vi "Robot Global Data.vi"() -> ()   [LabVIEW 2015]
doc: "This global VI can contain as many global variables as you need. Place a control on the panel, give it a good name. To read or write to it from a VI, drag the icon to the diagram of that VI. You can also drag from the project. Click on the node to change which global you access. You shouldn't have multiple locations writing to a global or it will cause a race-condition."
uses:
  <vilib>/Rock Robotics/WPI/Camera/WPI_CameraImageSize.ctl
  <vilib>/Rock Robotics/WPI/DriverStation/WPI_DriverStationRobotMode2.ctl
  Common Code/Auton Command Cluster.ctl
  Common Code/Drivetrain Status Cluster.ctl
  Common Code/Drivetrain Modes.ctl
  Common Code/Dist Drive Status.ctl
  Common Code/Dashboard Communication/Dashboard Display Data.ctl
  Common Code/Auton File Lists.ctl
  Common Code/Encoder Values Super Cluster.ctl
  Common Code/Encoder Values.ctl
  Common Code/IMU Data.ctl
  navX.Library.v2/navX Library v2/TypeDefs/Flags/Z900_navX_Flags_CalibrationStatusTypeDef.ctl
  navX.Library.v2/navX Library v2/TypeDefs/Flags/Z900_navX_Flags_OpStatusTypeDef.ctl
  Common Code/Power and Diagnostic Data.ctl
  Common Code/Utilities/PDP Data.ctl
  Common Code/Utilities/PCM Data.ctl
  Common Code/Intake Status Cluster.ctl
  Common Code/Intake Mode.ctl
  Common Code/Intake Commands.ctl
  Common Code/Ultrasonic Data.ctl
  Common Code/Major Loop Times.ctl
  Common Code/Catapult/Catapult Status Cluster.ctl
  Common Code/Catapult/Catapult Modes.ctl
  Common Code/Catapult/Catapult Auto Commands.ctl
  Common Code/Catapult/Shoot Mode.ctl
  Common Code/Dashboard Communication/Dashboard Control Data.ctl
  Common Code/Encoder Control.ctl
  Common Code/Drivetrain Settings.ctl
  Common Code/Goal Vision Packet.ctl
  Common Code/Dashboard Drivetrain Command.ctl
  Common Code/Drivetrain Vision.ctl
  Common Code/Ball Tracking Command Cluster.ctl
  Common Code/Ball Vision Packet.ctl
  Common Code/Tracking Mode.ctl
  Common Code/Intake Presets.ctl
  Common Code/Drivetrain Output Range.ctl
  Common Code/IntakeEcoderControl.ctl
  Common Code/Enabled Systems.ctl
  Common Code/Autonomous Presets.ctl
  Common Code/Auto Shift Cluster.ctl
  Common Code/Catapult/Catapult Presets.ctl
  Common Code/Climb Presets.ctl
  Common Code/Drivetrain Commands.ctl
  Common Code/Manual Shoot.ctl
  Common Code/Intake Commands Cluster.ctl
  Common Code/Manual Intake Commands.ctl
  Common Code/Keyboard Packet.ctl
  Common Code/Catapult/Catapult Command Cluster.ctl
  navX.Library.v2/navX Library v2/navX Library v2.lvlib
panel:
  in  "Catapult Status Cluster":T1={"Shoot? "=FALSE, "Mode"=enum."Auto", "States"=enum."Shoot", "Shoot Mode"=enum."Outer", "Override IR "=FALSE, "Ball Loaded? "=FALSE, "High Pressure?"=FALSE, "Enough Pressure? "=enum."NO ", "high 1"=FALSE, "high 2 "=FALSE, "high 3"=FALSE, "high 4"=FALSE, "Jank Boi"=FALSE, "Ball Security"=FALSE, "Flashlight "=FALSE}
  in  "Catapult Command Cluster":T5={"States"=enum."Shoot", "Mode"=enum."Auto", "Override IR"=FALSE, "Shoot Mode"=enum."Outer", "Ball Loaded?"=FALSE, "High Pressure?"=FALSE, "Shoot?"=FALSE, "Flashlight "=FALSE}
  in  "Goal Vision Packet":T6
  in  "Auton Line Number":i32
  out "Current Position":dbl
  out "Backward Intake Tripped?":bool
  out "Forward Intake Tripped?":bool
  in  "Zero Intake?":bool
  out "Auton File Loop Timer":u32
  out "US Loop Timer":u32
  out "Intake Loop Timer":u32
  out "Shooter Loop Timer":u32
  out "DT Loop Timer":u32
  out "Ultrasonic Data":T7
  in  "Keyboard Cluster":T8
  in  "Intake Status Cluster":T9={"Roller Power"=0.0, "Angle Power"=0.0, "Intake Mode"=enum."Auto", "Rollers Active?"=FALSE, "Current Height"=0.0, "Target Height"=0.0, "Encoder Raw Position"=0.0, "Forward Tripped?"=FALSE, "Backward Tripped?"=FALSE, "Override IR?"=FALSE, "Intake State"=enum."Zero"}
  out "Is IMU Reset?":bool
  in  "Reset IMU":bool
  in  "Boolean":bool
  in  "Intake Commands Cluster":T12={"Intake Commands"=enum."Load", "Intake Mode"=enum."Auto", "Override IR"=FALSE}
  in  "Manual Intake Commands":T13
  in  "Queue File Names":string[](array[string])
  in  "NavX Opened":bool
  in  "IMU Yaw Zero":dbl
  in  "IMU Roll Zero":dbl
  in  "IMU Pitch Zero":dbl
  in  "Manual Shoot":T14
  out "IMU Data":T15 {"OP Status" items=["INITIALIZING", "SELFTEST_IN_PROGRESS", "ERROR", "IMU_AUTOCAL_IN_PROGRESS", "NORMAL"]; "Calibration Status" items=["IMU_CAL_STATE_MASK"=3, "IMU_CAL_STATE_INPROGRESS"=0, "IMU_CAL_STATE_ACCUMULATE"=1, "IMU_CAL_STATE_COMPLETE"=2]}
  in  "Right Pot 0":dbl
  in  "Left Pot 0":dbl
  out "Encoder Values":T18
  in  "Dashboard Drivetrain Command":T20
  out "General Scripts":string
  in  "Auton File Lists":T22
  in  "Current Auton Command Data":T23
  in  "Dashboard Packet":T24={"Encoder Control"={"Right Tick Constant"=0.0, "Left Tick Constant"=0.0, "Reset?"=FALSE, "Y Dist"={"PID gains"={"proportional gain (Kc)"=0.0, "integral time (Ti, min)"=0.0, "derivative time (Td, min)"=0.0}}, "Y Stop Thresh"=0.0, "Y Stop Speed"=0.0}, "Steer PID output"={"output high"=0.0, "output low"=0.0}, " Steer PID gains"={"proportional gain (Kc)"=0.0, "integral time (Ti, min)"=0.0, "derivative time (Td, min)"=0.0}, "Drivetrain Settings"={"Gyro Tolerance"=0.0, "Throttle Ramp (ms)"=0.0, "Kv"=0.0, "Ka"=0.0, "Feed Forward P"=0.0, "Feed Forward D"=0.0, "Goal Vision PID gains"={"proportional gain (Kc)"=1.0, "integral time (Ti, min)"=0.01, "derivative time (Td, min)"=0.0}, "Goal Detection Window"=0.0, "Creep Rate"=0.0, "Vision Throttle Threshold"=0.0, "Min Turn Output"=0.0, "Left Batter Angle"=0.0, "Right Batter Angle"=0.0}, "Vision Packet"={"Distance"=0.0, "Center X"=0.0, "Center Y"=0.0, "Found Target?"=FALSE, "Robot Center"=0.0, "Angle"=0.0}, "Dashboard Drivetrain Command"={"Drivetrain Vision"={"Goal Window"=0.0, "Ball Window"=0.0}}, "Info/Command Cluster"={"Distance to Ball"=0.0, "Desired Angle"=0.0, "Command"=enum."Turn to Ball", "Pixels from Center"=0.0}, "Ball Vision Packet"={"Ball Detected?"=FALSE, "Distance to Ball"=0.0, "Desired Angle"=0.0, "Pixels from Center"=0.0, "Tracking mode"=enum."Turn to Ball"}, "Intake Presets"={"Intake Speed"=0.0, "Outake Speed"=0.0, "Angle Speed"=0.0, "Angle Tolerance"=0.0, "Encoder Scale"=0.0, "Load Height"=0.0, "Output Range"={"output high"=0.0, "output low"=0.0}, "MaxCurrent"=0.0, "Idle Height"=0.0, "Max Height"=0.0, "Reset Encoders?"=FALSE, "PID gains"={"proportional gain (Kc)"=0.0, "integral time (Ti, min)"=0.0, "derivative time (Td, min)"=0.0}, "Drop Low Height "=0.0, "Rotation Power Max/Min"=0.0, "Reset Delay"=0.0}, "Intake Encoder Control"={"Arm Tick Constant"=0.0, "Reset?"=FALSE, "Y Dist"={"PID gains"={"proportional gain (Kc)"=0.0, "integral time (Ti, min)"=0.0, "derivative time (Td, min)"=0.0}}, "Y Stop Thresh"=0.0, "Y Stop Speed"=0.0}, "Goal Output Range"={"output high"=0.0, "output low"=0.0}, "Enabled Systems"={"Shoot"=TRUE, "Intake"=TRUE, "DT"=TRUE, "Gyro"=TRUE, "100ms"=TRUE, "US"=TRUE}, "Auton Presets"={"Pitch Limit"=0.0, "Roll Limit"=0.0, "Start Position"=0.0, "Cross Position"=0.0}, "Pressure M"=0.0, "Pressure B"=0.0, "Vision Timeout"=0.0, "Auto-Shift"={"Delay"=0.0, "Speed Thresh"=0.0, "Upshift Accel"=0.0, "Upshift Throttle"=0.0, "Upshift Throttle Accel"=0.0, "Downshift Throttle"=0.0, "Downshift Throttle Accel"=0.0, "Pressure Threshold"=0.0}, "Catapult Setpoints"={"Intake Danger Height"=0.0, "Ball Security Delay "=0.0, "High PSI Minimum"=0.0, "Shot Finish Delay"=0.0, "Low PSI Minimum"=0.0, "Idle Ball Security Wait "=0.0}, "Climb Presets"={"Winch Speed"=0.0}} {"Intake Presets"."Reset Delay" format="%#_7g"; "Intake Presets"."Rotation Power Max/Min" format="%#_7g"; "Intake Presets"."Drop Low Height" format="%#_7g"; "Intake Presets"."Max Height" format="%#_7g"; "Drivetrain Settings"."Goal Vision PID gains"."derivative time (Td, min)" format="%.3f"; "Drivetrain Settings"."Goal Vision PID gains"."integral time (Ti, min)" format="%.3f"; "Drivetrain Settings"."Goal Vision PID gains"."proportional gain (Kc)" format="%.3f"}
  out "Driver Station IP":u32
  in  "Auton File Index":i32
  in  "Auton Field Index":i32
  out "Dashboard Status Data":T38={"Auton Command Cluster"={"Command ID"=0, "maxTime"=0.0, "Y Distance"=0.0, "Heading"=0.0, "Throttle"=0.0, "Async"=0.0, "Velocity"=0.0, "Acceleration"=0.0, "To"=0.0, "Condition"=0.0, "Shot Type"=0.0, "Left RPM"=0.0, "Override RPM"=0, "Override Angle"=0, "Right RPM"=0.0, "Angle"=0.0, "Intake Mode"=0, "Intake Cmd"=0, "Intake O"=0, "Eject O"=0, "Angle O"=0, "Arm O"=0, "Intake Speed"=0.0, "Eject Speed"=0.0, "Arm Angle"=0.0, "Arm Speed"=0.0, "Intake?"=0, "Eject?"=0, "Left"=0.0, "Right"=0.0, "Pivot Speed"=0.0, "Y Dist"=0.0, "Position"=0.0, "Desired Position"=0, "Shooter Mode"=0.0, "Shooter Command"=0.0, "Shoot?"=0.0, "Shoot mode"=0.0}, "Auton File Lists"={"Current Queue"="", "General Scripts"="", "Defense Scripts"="", "Movement Scripts"=""}, "Drivetrain Status Cluster"={"Modes"=enum."Manual", "Y (Throttle)"=0.0, "X (Steer)"=0.0, "Gyro In Range?"=FALSE, "Distance Drive Finished?"=FALSE, "Stop Eject Lockout"=FALSE, "Dist Drive Status"={"Y In Range"=FALSE, "X In Range"=FALSE, "Gyro In Range"=FALSE, "Y Dist"=0.0, "X Dist"=0.0, "Gyro"=0.0}, "Y Target"=0.0, "Heading Target"=0.0, "Vision Target Aligned?"=FALSE}, "Encoder Values"={"Left Encoder"={"Distance"=0.0, "Speed"=0.0, "Ticks"=0.0}, "Right Encoder"={"Distance"=0.0, "Speed"=0.0, "Ticks"=0.0}}, "IMU Data"={"Pitch"=0.0, "Roll"=0.0, "Yaw"=0.0, "Data Valid?"=FALSE, "Temp"=0.0, "MOVING"=FALSE, "YAW_STABLE"=FALSE, "Accel X"=0.0, "Accel Y"=0.0, "Accel Z"=0.0, "Accel Magnitude"=0.0, "Pitch Rate"=0.0, "Roll Rate"=0.0, "Yaw Rate"=0.0, "NavX Opened?"=FALSE, "Calibration Status"=0, "OP Status"=0}, "Power and Diagnostic Data"={"PDP Data"={"Battery Voltage"=0.0, "Temperature (degrees C)"=0.0, "Internal Battery R (Ohms)"=0.0, "Energy (J)"=0.0, "Power (W)"=0.0, "Total Current (A)"=0.0, "Battery Voltage Fault"=FALSE, "Temperature Fault"=FALSE, "Hardware Fault"=FALSE, "Currents"={"[0]"=0.0, "[1]"=0.0, "[2]"=0.0, "[3]"=0.0, "[4]"=0.0, "[5]"=0.0, "[6]"=0.0, "[7]"=0.0, "[8]"=0.0, "[9]"=0.0, "[10]"=0.0, "[11]"=0.0, "[12]"=0.0, "[13]"=0.0, "[14]"=0.0, "[15]"=0.0}, "Current Faults"={"[0]"=FALSE, "[1]"=FALSE, "[2]"=FALSE, "[3]"=FALSE, "[4]"=FALSE, "[5]"=FALSE, "[6]"=FALSE, "[7]"=FALSE, "[8]"=FALSE, "[9]"=FALSE, "[10]"=FALSE, "[11]"=FALSE, "[12]"=FALSE, "[13]"=FALSE, "[14]"=FALSE, "[15]"=FALSE}}, "PCM Data"={"Compressor Fault"=FALSE, "Solenoid Fault"=FALSE, "Compressor Enabled"=FALSE, "Hardware Fault"=FALSE, "Compressor Current"=0.0}, "roboRIO input voltage (V)"=0.0, "roboRIO input current (A)"=0.0, "3.3V Rail Short"=FALSE, "5 V Rail Short"=FALSE, "6 V Rail Short"=FALSE, "roboRIO Brownout"=FALSE, "Outputs Enabled?"=FALSE}, "Gyro"=0.0, "Intake Status Cluster"={"Roller Power"=0.0, "Angle Power"=0.0, "Intake Mode"=enum."Auto", "Rollers Active?"=FALSE, "Current Height"=0.0, "Target Height"=0.0, "Encoder Raw Position"=0.0, "Forward Tripped?"=FALSE, "Backward Tripped?"=FALSE, "Override IR?"=FALSE, "Intake State"=enum."Zero"}, "Ultrasonic Data"={"Left Ultrasonic"=0.0, "Right Ultrasonic"=0.0}, "Loop Times"={"DT Loop Timer"=0, "Shooter Loop Timer"=0, "Intake Loop Timer"=0, "US Loop Timer"=0, "Auton File Loop Timer"=0}, "Pressure"=0.0, "Pressure Voltage"=0.0, "Auton Line Number"=0, "Catapult Status Cluster "={"Shoot? "=FALSE, "Mode"=enum."Auto", "States"=enum."Shoot", "Shoot Mode"=enum."Outer", "Override IR "=FALSE, "Ball Loaded? "=FALSE, "High Pressure?"=FALSE, "Enough Pressure? "=enum."NO ", "high 1"=FALSE, "high 2 "=FALSE, "high 3"=FALSE, "high 4"=FALSE, "Jank Boi"=FALSE, "Ball Security"=FALSE, "Flashlight "=FALSE}, "Forward Tripped?"=FALSE, "Backward Tripped?"=FALSE} {"IMU Data"."OP Status" items=["INITIALIZING", "SELFTEST_IN_PROGRESS", "ERROR", "IMU_AUTOCAL_IN_PROGRESS", "NORMAL"]; "IMU Data"."Calibration Status" items=["IMU_CAL_STATE_MASK"=3, "IMU_CAL_STATE_INPROGRESS"=0, "IMU_CAL_STATE_ACCUMULATE"=1, "IMU_CAL_STATE_COMPLETE"=2]}
  in  "Auton File Build Loops":i32
  in  "Auton File Queue":path[](array[path])
  in  "Auton Command Array":T23[](array[typedef])
  out "Drivetrain Status Cluster":T39={"Modes"=enum."Manual", "Y (Throttle)"=0.0, "X (Steer)"=0.0, "Gyro In Range?"=FALSE, "Distance Drive Finished?"=FALSE, "Stop Eject Lockout"=FALSE, "Dist Drive Status"={"Y In Range"=FALSE, "X In Range"=FALSE, "Gyro In Range"=FALSE, "Y Dist"=0.0, "X Dist"=0.0, "Gyro"=0.0}, "Y Target"=0.0, "Heading Target"=0.0, "Vision Target Aligned?"=FALSE}
  in  "Drivetrain Command Cluster":T46={"Y Power"=0.0, "Turn Power"=0.0, "Modes"=enum."Manual", "Heading Target"=0.0, "X Max Speed"=0.0, "Y Max Speed"=0.0, "X Min Speed"=0.0, "Y Min Speed"=0.0, "Y Target"=0.0, "Max Accel"=0.0, "Max Velocity"=0.0, "Pivot Speed"=0.0}
  in  "Robot Mode":T47
  in  "image size":T48=enum."320x240"
  in  "Enable Vision":bool
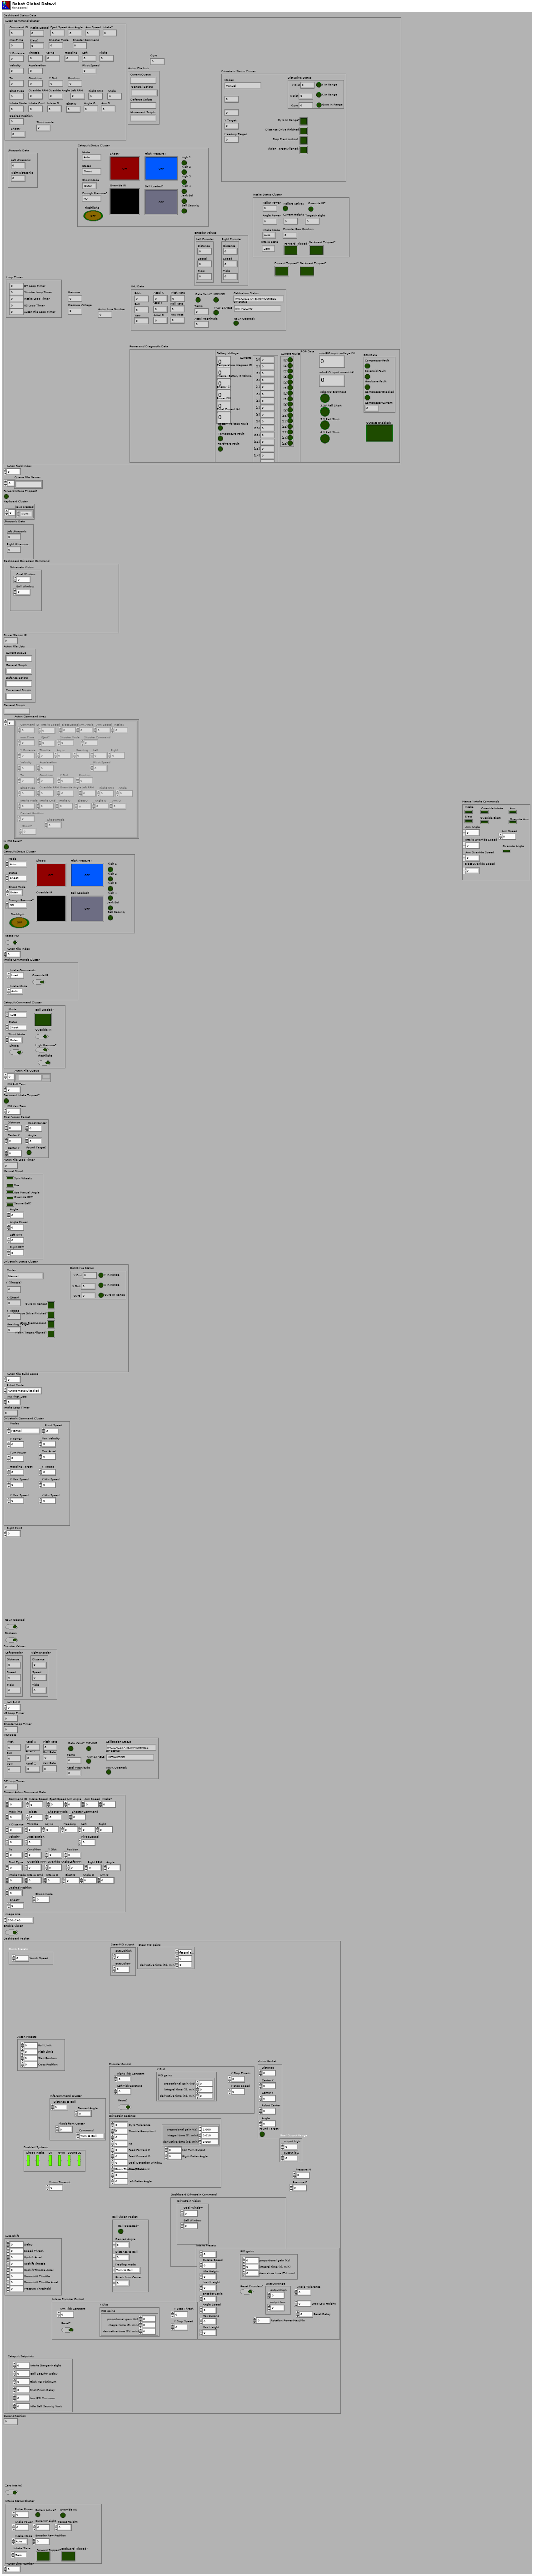
[diagram p1: front panel]
types:
  T1 = typedef "Catapult Status Cluster.ctl" = cluster{"Shoot? ":bool, "Mode":T2, "States":T3, "Shoot Mode":T4, "Override IR ":bool, "Ball Loaded? ":bool, "High Pressure?":bool, "Enough Pressure? ":enum16{"NO ", "Low Pressure", "High Pressure "}, "high 1":bool, "high 2 ":bool, "high 3":bool, "high 4":bool, "Jank Boi":bool, "Ball Security":bool, "Flashlight ":bool}
  T2 = typedef "Catapult Modes.ctl" = enum16{"Auto"}
  T3 = typedef "Catapult Auto Commands.ctl" = enum16{"Idle", "Warmup", "Shoot"}
  T4 = typedef "Shoot Mode.ctl" = enum16{"Outer", "Batter"}
  T5 = typedef "Catapult Command Cluster.ctl" = cluster{"States":T3, "Mode":T2, "Override IR":bool, "Shoot Mode":T4, "Ball Loaded?":bool, "High Pressure?":bool, "Shoot?":bool, "Flashlight ":bool}
  T6 = typedef "Goal Vision Packet.ctl" = cluster{"Distance":dbl, "Center X":dbl, "Center Y":dbl, "Found Target?":bool, "Robot Center":dbl, "Angle":dbl}
  T7 = typedef "Ultrasonic Data.ctl" = cluster{"Left Ultrasonic":dbl, "Right Ultrasonic":dbl}
  T8 = typedef "Keyboard Packet.ctl" = cluster{"keys pressed":enum16{"0", "1", "2", "3", "4", "5", "6", "7", "8", "9", "A", "B", "C", "D", "E", "F", "G", "H", "I", "J", "K", "L", "M", "N", "O", "P", "Q", "R", "S", "T", "U", "V", "W", "X", "Y", "Z", "F1", "F2", "F3", "F4", "F5", "F6", "F7", "F8", "F9", "F10", "F11", "F12", "F13", "F14", "F15", "ADD", "BACK", "BACKSLASH", "CAPITAL", "COMMA", "DECIMAL", "DELETE", "DIVIDE", "DOWN", "END", "EQUALS", "ESCAPE", "GRAVE (`)", "HOME", "INSERT", "LBRACKET", "LCONTROL", "LEFT", "L ALT", "LSHIFT", "LWIN", "MINUS", "MULTIPLY", "NEXT", "NUMLOCK", "NUMPAD_0", "NUMPAD_1", "NUMPAD_2", "NUMPAD_3", "NUMPAD_4", "NUMPAD_5", "NUMPAD_6", "NUMPAD_7", "NUMPAD_8", "NUMPAD_9", "PAUSE", "PERIOD", "PRIOR (PG UP)", "RBRACKET", "RCONTROL", "RETURN", "RIGHT", "R ALT", "RSHIFT", "RWIN", "SCROLL", "SEMICOLON", "SLASH", "SPACE", "SUBTRACT", "TAB", "UP", "ENTER (num pad)", "' (quote)"}[]}
  T9 = typedef "Intake Status Cluster.ctl" = cluster{"Roller Power":dbl, "Angle Power":dbl, "Intake Mode":T10, "Rollers Active?":bool, "Current Height":dbl, "Target Height":dbl, "Encoder Raw Position":dbl, "Forward Tripped?":bool, "Backward Tripped?":bool, "Override IR?":bool, "Intake State":T11}
  T10 = typedef "Intake Mode.ctl" = enum16{"Manual", "Safe", "Auto"}
  T11 = typedef "Intake Commands.ctl" = enum16{"Zero", "Unload", "Load", "Drop low", "Idle"}
  T12 = typedef "Intake Commands Cluster.ctl" = cluster{"Intake Commands":T11, "Intake Mode":T10, "Override IR":bool}
  T13 = typedef "Manual Intake Commands.ctl" = cluster{"Intake":bool, "Eject":bool, "Arm Angle":dbl, "Intake Override Speed":dbl, "Arm Override Speed":dbl, "Arm Speed":dbl, "Override Intake":bool, "Override Eject":bool, "Eject Override Speed":dbl, "Arm":bool, "Override Arm":bool, "Override Angle":bool}
  T14 = typedef "Manual Shoot.ctl" = cluster{"Spin Wheels":bool, "Fire":bool, "Angle":dbl, "Angle Power":dbl, "Use Manual Angle":bool, "Override RPM":bool, "Left RPM":dbl, "Right RPM":dbl, "Secure Ball?":bool}
  T15 = typedef "IMU Data.ctl" = cluster{"Pitch":sgl, "Roll":sgl, "Yaw":sgl, "Data Valid?":bool, "Temp":sgl, "MOVING":bool, "YAW_STABLE":bool, "Accel X":sgl, "Accel Y":sgl, "Accel Z":sgl, "Accel Magnitude":sgl, "Pitch Rate":sgl, "Roll Rate":sgl, "Yaw Rate":sgl, "NavX Opened?":bool, "Calibration Status":T16, "OP Status":T17}
  T16 = typedef "navX Library v2.lvlib/Z900_navX_Flags_CalibrationStatusTypeDef.ctl" = u8
  T17 = typedef "navX Library v2.lvlib/Z900_navX_Flags_OpStatusTypeDef.ctl" = u8
  T18 = typedef "Encoder Values Super Cluster.ctl" = cluster{"Left Encoder":T19, "Right Encoder":T19}
  T19 = typedef "Encoder Values.ctl" = cluster{"Distance":dbl, "Speed":dbl, "Ticks":dbl}
  T20 = typedef "Dashboard Drivetrain Command.ctl" = cluster{"Drivetrain Vision":T21}
  T21 = typedef "Drivetrain Vision.ctl" = cluster{"Goal Window":dbl, "Ball Window":dbl}
  T22 = typedef "Auton File Lists.ctl" = cluster{"Current Queue":string, "General Scripts":string, "Defense Scripts":string, "Movement Scripts":string}
  T23 = typedef "Auton Command Cluster.ctl" = cluster{"Command ID":i32, "maxTime":dbl, "Y Distance":dbl, "Heading":dbl, "Throttle":dbl, "Async":dbl, "Velocity":dbl, "Acceleration":dbl, "To":dbl, "Condition":dbl, "Shot Type":dbl, "Left RPM":dbl, "Override RPM":i32, "Override Angle":i32, "Right RPM":dbl, "Angle":dbl, "Intake Mode":i32, "Intake Cmd":i32, "Intake O":i32, "Eject O":i32, "Angle O":i32, "Arm O":i32, "Intake Speed":dbl, "Eject Speed":dbl, "Arm Angle":dbl, "Arm Speed":dbl, "Intake?":i32, "Eject?":i32, "Left":dbl, "Right":dbl, "Pivot Speed":dbl, "Y Dist":dbl, "Position":dbl, "Desired Position":i32, "Shooter Mode":dbl, "Shooter Command":dbl, "Shoot?":dbl, "Shoot mode":dbl}
  T24 = typedef "Dashboard Control Data.ctl" = cluster{"Encoder Control":T25, "Steer PID output":cluster{"output high":dbl, "output low":dbl}, " Steer PID gains":cluster{"proportional gain (Kc)":dbl, "integral time (Ti, min)":dbl, "derivative time (Td, min)":dbl}, "Drivetrain Settings":T26, "Vision Packet":T6, "Dashboard Drivetrain Command":T20, "Info/Command Cluster":T27, "Ball Vision Packet":T28, "Intake Presets":T30, "Intake Encoder Control":T32, "Goal Output Range":cluster{"output high":dbl, "output low":dbl}, "Enabled Systems":T33, "Auton Presets":T34, "Pressure M":dbl, "Pressure B":dbl, "Vision Timeout":dbl, "Auto-Shift":T35, "Catapult Setpoints":T36, "Climb Presets":T37}
  T25 = typedef "Encoder Control.ctl" = cluster{"Right Tick Constant":dbl, "Left Tick Constant":dbl, "Reset?":bool, "Y Dist":cluster{"PID gains":cluster{"proportional gain (Kc)":dbl, "integral time (Ti, min)":dbl, "derivative time (Td, min)":dbl}}, "Y Stop Thresh":dbl, "Y Stop Speed":dbl}
  T26 = typedef "Drivetrain Settings.ctl" = cluster{"Gyro Tolerance":dbl, "Throttle Ramp (ms)":dbl, "Kv":dbl, "Ka":dbl, "Feed Forward P":dbl, "Feed Forward D":dbl, "Goal Vision PID gains":cluster{"proportional gain (Kc)":dbl, "integral time (Ti, min)":dbl, "derivative time (Td, min)":dbl}, "Goal Detection Window":dbl, "Creep Rate":dbl, "Vision Throttle Threshold":dbl, "Min Turn Output":dbl, "Left Batter Angle":dbl, "Right Batter Angle":dbl}
  T27 = typedef "Ball Tracking Command Cluster.ctl" = cluster{"Distance to Ball":dbl, "Desired Angle":dbl, "Command":enum16{"Turn to Ball", "Turn to Angle", "Get Distance"}, "Pixels from Center":dbl}
  T28 = typedef "Ball Vision Packet.ctl" = cluster{"Ball Detected?":bool, "Distance to Ball":dbl, "Desired Angle":dbl, "Pixels from Center":dbl, "Tracking mode":T29}
  T29 = typedef "Tracking Mode.ctl" = enum16{"Turn to Ball", "Turn to Angle"}
  T30 = typedef "Intake Presets.ctl" = cluster{"Intake Speed":dbl, "Outake Speed":dbl, "Angle Speed":dbl, "Angle Tolerance":dbl, "Encoder Scale":dbl, "Load Height":dbl, "Output Range":T31, "MaxCurrent":dbl, "Idle Height":dbl, "Max Height":dbl, "Reset Encoders?":bool, "PID gains":cluster{"proportional gain (Kc)":dbl, "integral time (Ti, min)":dbl, "derivative time (Td, min)":dbl}, "Drop Low Height ":dbl, "Rotation Power Max/Min":dbl, "Reset Delay":dbl}
  T31 = typedef "Drivetrain Output Range.ctl" = cluster{"output high":dbl, "output low":dbl}
  T32 = typedef "IntakeEcoderControl.ctl" = cluster{"Arm Tick Constant":dbl, "Reset?":bool, "Y Dist":cluster{"PID gains":cluster{"proportional gain (Kc)":dbl, "integral time (Ti, min)":dbl, "derivative time (Td, min)":dbl}}, "Y Stop Thresh":dbl, "Y Stop Speed":dbl}
  T33 = typedef "Enabled Systems.ctl" = cluster{"Shoot":bool, "Intake":bool, "DT":bool, "Gyro":bool, "100ms":bool, "US":bool}
  T34 = typedef "Autonomous Presets.ctl" = cluster{"Pitch Limit":dbl, "Roll Limit":dbl, "Start Position":dbl, "Cross Position":dbl}
  T35 = typedef "Auto Shift Cluster.ctl" = cluster{"Delay":dbl, "Speed Thresh":dbl, "Upshift Accel":dbl, "Upshift Throttle":dbl, "Upshift Throttle Accel":dbl, "Downshift Throttle":dbl, "Downshift Throttle Accel":dbl, "Pressure Threshold":dbl}
  T36 = typedef "Catapult Presets.ctl" = cluster{"Intake Danger Height":dbl, "Ball Security Delay ":dbl, "High PSI Minimum":dbl, "Shot Finish Delay":dbl, "Low PSI Minimum":dbl, "Idle Ball Security Wait ":dbl}
  T37 = typedef "Climb Presets.ctl" = cluster{"Winch Speed":dbl}
  T38 = typedef "Dashboard Display Data.ctl" = cluster{"Auton Command Cluster":T23, "Auton File Lists":T22, "Drivetrain Status Cluster":T39, "Encoder Values":T18, "IMU Data":T15, "Power and Diagnostic Data":T42, "Gyro":dbl, "Intake Status Cluster":T9, "Ultrasonic Data":T7, "Loop Times":T45, "Pressure":dbl, "Pressure Voltage":dbl, "Auton Line Number":i32, "Catapult Status Cluster ":T1, "Forward Tripped?":bool, "Backward Tripped?":bool}
  T39 = typedef "Drivetrain Status Cluster.ctl" = cluster{"Modes":T40, "Y (Throttle)":dbl, "X (Steer)":dbl, "Gyro In Range?":bool, "Distance Drive Finished?":bool, "Stop Eject Lockout":bool, "Dist Drive Status":T41, "Y Target":dbl, "Heading Target":dbl, "Vision Target Aligned?":bool}
  T40 = typedef "Drivetrain Modes.ctl" = enum16{"Gyro Steer", "Manual", "Goal Vision Targeting", "PID Distance Drive", "Hybrid"}
  T41 = typedef "Dist Drive Status.ctl" = cluster{"Y In Range":bool, "X In Range":bool, "Gyro In Range":bool, "Y Dist":dbl, "X Dist":dbl, "Gyro":dbl}
  T42 = typedef "Power and Diagnostic Data.ctl" = cluster{"PDP Data":T43, "PCM Data":T44, "roboRIO input voltage (V)":dbl, "roboRIO input current (A)":dbl, "3.3V Rail Short":bool, "5 V Rail Short":bool, "6 V Rail Short":bool, "roboRIO Brownout":bool, "Outputs Enabled?":bool}
  T43 = typedef "PDP Data.ctl" = cluster{"Battery Voltage":sgl, "Temperature (degrees C)":sgl, "Internal Battery R (Ohms)":sgl, "Energy (J)":sgl, "Power (W)":sgl, "Total Current (A)":sgl, "Battery Voltage Fault":bool, "Temperature Fault":bool, "Hardware Fault":bool, "Currents":cluster{"[0]":sgl, "[1]":sgl, "[2]":sgl, "[3]":sgl, "[4]":sgl, "[5]":sgl, "[6]":sgl, "[7]":sgl, "[8]":sgl, "[9]":sgl, "[10]":sgl, "[11]":sgl, "[12]":sgl, "[13]":sgl, "[14]":sgl, "[15]":sgl}, "Current Faults":cluster{"[0]":bool, "[1]":bool, "[2]":bool, "[3]":bool, "[4]":bool, "[5]":bool, "[6]":bool, "[7]":bool, "[8]":bool, "[9]":bool, "[10]":bool, "[11]":bool, "[12]":bool, "[13]":bool, "[14]":bool, "[15]":bool}}
  T44 = typedef "PCM Data.ctl" = cluster{"Compressor Fault":bool, "Solenoid Fault":bool, "Compressor Enabled":bool, "Hardware Fault":bool, "Compressor Current":dbl}
  T45 = typedef "Major Loop Times.ctl" = cluster{"DT Loop Timer":u32, "Shooter Loop Timer":u32, "Intake Loop Timer":u32, "US Loop Timer":u32, "Auton File Loop Timer":u32}
  T46 = typedef "Drivetrain Commands.ctl" = cluster{"Y Power":dbl, "Turn Power":dbl, "Modes":T40, "Heading Target":dbl, "X Max Speed":dbl, "Y Max Speed":dbl, "X Min Speed":dbl, "Y Min Speed":dbl, "Y Target":dbl, "Max Accel":dbl, "Max Velocity":dbl, "Pivot Speed":dbl}
  T47 = typedef "WPI_DriverStationRobotMode2.ctl" = enum16{"Autonomous Disabled", "Autonomous Enabled", "Teleop Disabled", "Teleop Enabled", "Disconnected", "Finish", "Test Disabled", "Test Enabled", "Emergency Stopped"}
  T48 = typedef "WPI_CameraImageSize.ctl" = enum16{"640x480", "320x240", "160x120", "Custom"}
diagram:
